vi "extract Pan value(SubVI).vi"(6 "0.1/0/01":bool, 8 "error in (no error)":errorcluster, 9 "TimeOut":bool, 11 "response":string) -> (0 "error out":errorcluster, 3 "pan angle":dbl format="%.2f")   [LabVIEW 2018]
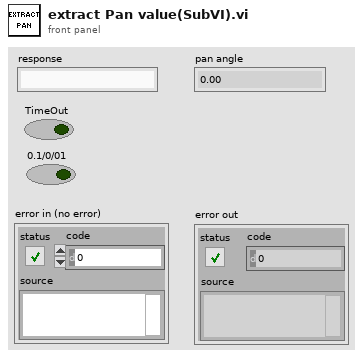
[diagram p1: front panel]
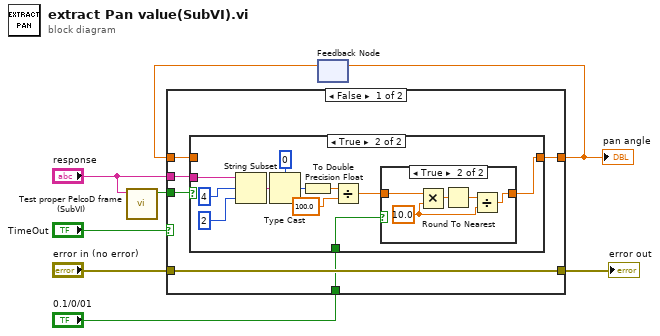
[diagram p0: block diagram]
diagram:
  n1 = call "Test proper PelcoD frame (SubVI).vi"("Pelco-D frame"="response") -> ("Proper?"=w2:bool)  [unwired: 10 in]
  n2 = feedback #1() -> (w4:dbl)  [unwired: 1 in]
  n3 = case shown="False" "TimeOut" {
    tunnel: "error in (no error)" -> [w14 w33]
    tunnel: [w14 w33] -> w6
    tunnel: [w13 w34] -> w5
    tunnel: w4 -> [w12 w34]
    tunnel: "0.1/0/01" -> [w11 _]
    tunnel: w2 -> [w10 _]
    tunnel: "response" -> [w9 _]
    frame False {
      n4 = case shown="True" w10 {
        tunnel: w9 -> [_ w21]
        tunnel: [w15 w19] -> w13
        tunnel: w12 -> [w15 _]
        tunnel: w11 -> [_ w16]
        frame False {
        }
        frame True {
          n5 = String Subset(string=w21, offset (0)=4, length (rest)=2 ("length (rest)")) -> (substring=w25:string)
          n6 = Type Cast(type=u16 0, x=w25) -> (*(type *) &x=w18:u16)
          n7 = To Double Precision Float(number=w18) -> (double precision float=w17:dbl)
          n8 = Divide(x=w17, y=100.0) -> (x/y=w20:dbl)
          n9 = case shown="True" w16 {
            tunnel: w20 -> [w27 w29]
            tunnel: [w27 w28] -> w19
            frame False {
            }
            frame True {
              w30 = 10.0
              n10 = Multiply(x=w29, y=w30) -> (x*y=w32:dbl)
              n11 = Round To Nearest(number=w32) -> (nearest integer value=w31:dbl)
              n12 = Divide(x=w31, y=w30) -> (x/y=w28:dbl)
            }
          }
        }
      }
    }
    frame True {
    }
  }
  "error out" <- w6
  "pan angle" <- w5
  n13 = feedback-in #1(w5) -> ()
